vi "Read Value.vi"(8 "error in (no error)":errorcluster, 11 "fixed64 in":refnum<class "fixed64.lvclass">) -> (0 "error out":errorcluster, 2 "Value":u64, 3 "fixed64 out":refnum<class "fixed64.lvclass">)   [LabVIEW 2020, in "Protobuf RAW.lvlib" / "fixed64.lvclass"]
uses:
  fixed64.lvclass
  fixed64.lvclass/fixed64.ctl
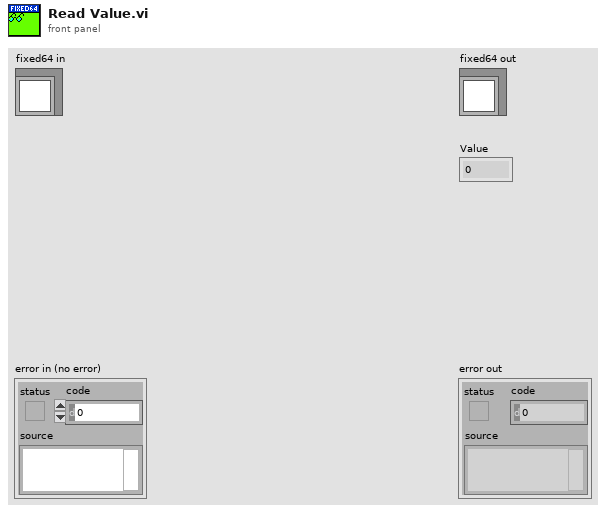
[diagram p1: front panel]
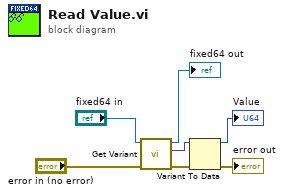
[diagram p0: block diagram]
diagram:
  n1 = call-dynamic "Get Variant.vi"("error in (no error)"="error in (no error)", "int32 in"="fixed64 in") -> ("error out"=w6:errorcluster, "Variant"=w2:variant, "int32 out"=→"fixed64 out":refnum<class "fixed64.lvclass">)  [unwired: 7 in]
  n2 = Variant To Data(error in=w6, Variant=w2) -> (data=→"Value":u64, error out=→"error out":errorcluster)  [unwired: 1 in]
